vi "controlFrequency.vi"(7 "Set":bool, 8 "error in":errorcluster, 9 "Frequenzy [Hz] in":dbl, 10 "axis in":u8, 11 "connection ID":i32) -> (0 "error out":errorcluster, 1 "Frequenzy [Hz] out":dbl, 2 "axis out":u8, 3 "connection ID":i32)   [LabVIEW 2016]
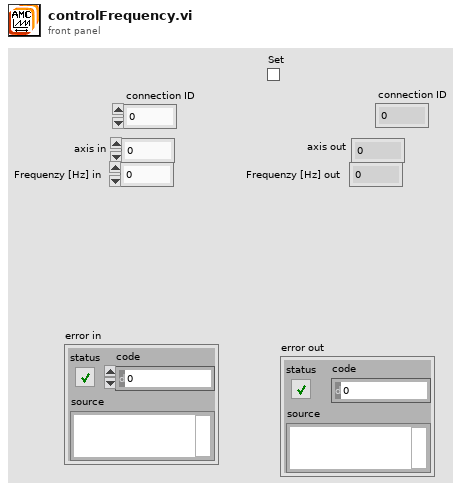
[diagram p1: front panel]
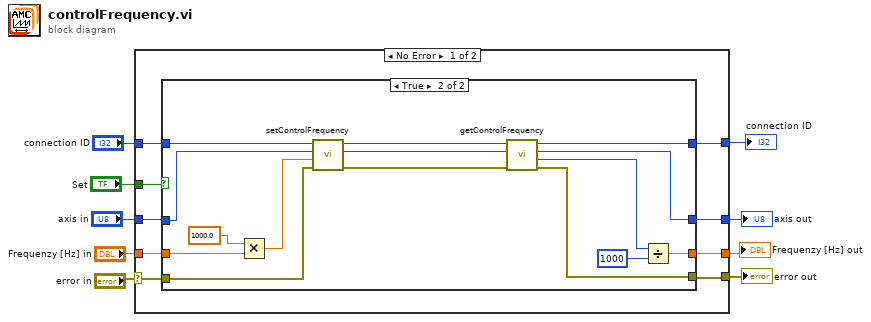
[diagram p0: block diagram]
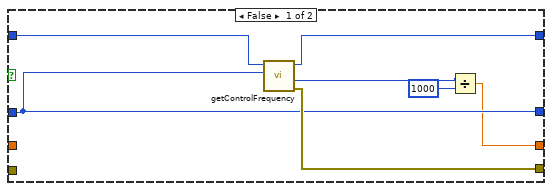
[diagram p2: hidden frame]
diagram:
  n1 = case shown="No Error" "error in" {
    selector: "error in" -> [w14 w44]
    tunnel: "axis in" -> [w16 w42]
    tunnel: [w10 w44] -> w8
    tunnel: [w12 w42] -> w7
    tunnel: "Frequenzy [Hz] in" -> [w15 w43]
    tunnel: [w11 w43] -> w5
    tunnel: "Set" -> [w17 _]
    tunnel: [w13 w41] -> w3
    tunnel: "connection ID" -> [w18 w41]
    frame No Error {
      n2 = case shown="True" w17 {
        tunnel: [w24 w34] -> w13
        tunnel: w18 -> [w25 w40]
        tunnel: w16 -> [w22 w28]
        tunnel: [w22 w26] -> w12
        tunnel: [w23 w31] -> w10
        tunnel: [w19 w29] -> w11
        tunnel: w15 -> [_ w38]
        tunnel: w14 -> [_ w36]
        frame False {
          n3 = call "getControlFrequency.vi"("axis"=w22, "connection ID"=w25) -> ("error out"=w23:errorcluster, "frequency"=w21:i32, "connection ID"=w24:i32)  [unwired: 6 in, 1 out]
          n4 = Divide(x=w21, y=1000) -> (x/y=w19:dbl)
        }
        frame True {
          n5 = Multiply(x=1000.0, y=w38) -> (x*y=w37:dbl)
          n6 = call "setControlFrequency.vi"("error in"=w36, "frequency"=w37, "axis"=w28, "connection ID"=w40) -> ("error out"=w32:errorcluster, "axis_out"=w27:i32, "connection ID"=w35:i32)  [unwired: 5 in]
          n7 = call "getControlFrequency.vi"("error in"=w32, "axis"=w27, "connection ID"=w35) -> ("error out"=w31:errorcluster, "frequency"=w30:i32, "axis_out"=w26:i32, "connection ID"=w34:i32)  [unwired: 5 in]
          n8 = Divide(x=w30, y=1000) -> (x/y=w29:dbl)
        }
      }
    }
    frame Error {
    }
  }
  "error out" <- w8
  "axis out" <- w7
  "Frequenzy [Hz] out" <- w5
  "connection ID" <- w3
